vi "Example Circular Buffer Map.vi"() -> ()   [LabVIEW 2013]
uses:
  VariantBuffer/VariantBuffer.lvclass
  VariantBufferMap/VariantBufferMap.lvclass
panel:
  out "error out":errorcluster
  in  "preview count (-1: all)":i32=5
  out "found":bool
  out "elements":variant[](array[variant])
  in  "Buffer Name":string(combo)
  # "Select the Buffer to Preview"
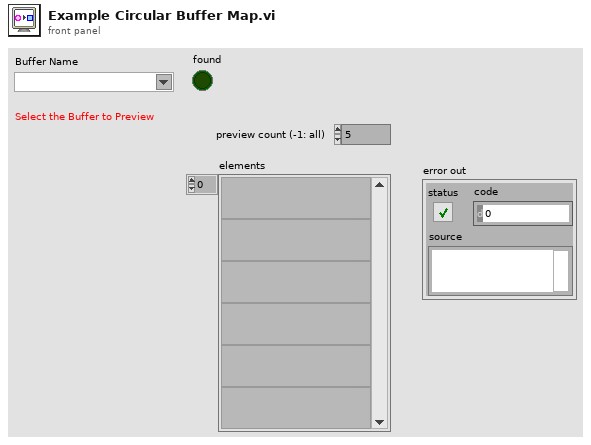
[diagram p1: front panel]
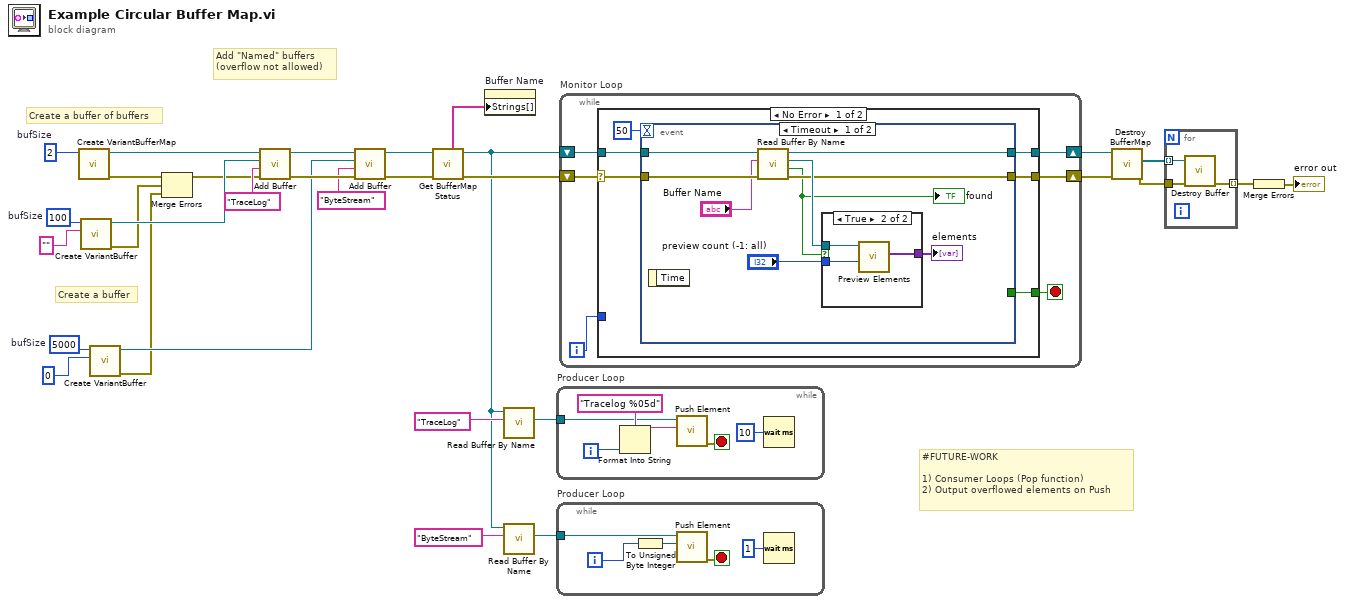
[diagram p0: block diagram]
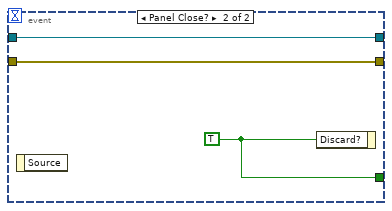
[diagram p3: hidden frame]
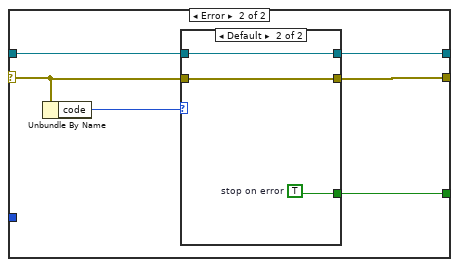
[diagram p4: hidden frame]
diagram:
  w8 = 5000  # bufSize
  w29 = 2  # bufSize
  w31 = 100  # bufSize
  # "#FUTURE-WORK\n\n1) Consumer Loops (Pop function)\n2) Output overflowed elements on Push"
  # "Create a buffer"
  # "Add \"Named\" buffers\n(overflow not allowed)"
  # "Create a buffer of buffers"
  n1 = call "Create VariantBufferMap.vi"("bufSize"=w29) -> ("error out"=w22:errorcluster, "BufferMap"=w23:refnum<data-value>)  [unwired: 9 in]
  n2 = call "Create VariantBuffer.vi"("default"="", "bufSize"=w31) -> ("error out"=w21:errorcluster, "Buffer"=w27:refnum<data-value>)  [unwired: 8 in]
  n3 = call "Create VariantBuffer.vi"("default"=u8 0, "bufSize"=w8) -> ("error out"=w4:errorcluster, "Buffer"=w6:refnum<data-value>)  [unwired: 8 in]
  n4 = Merge Errors(w22, w21, w4) -> (w20:errorcluster)
  n5 = call "Add Buffer.vi"("error in"=w20, "Name"="TraceLog", "Buffer"=w27, "BufferMap in"=w23) -> ("error out"=w11:errorcluster, "BufferMap"=w13:refnum<data-value>)  [unwired: 6 in]
  n6 = call "Add Buffer.vi"("error in"=w11, "Name"="ByteStream", "Buffer"=w6, "BufferMap in"=w13) -> ("error out"=w10:errorcluster, "BufferMap"=w12:refnum<data-value>)  [unwired: 6 in]
  n7 = call "Get BufferMap Status.vi"("error in"=w10, "BufferMap in"=w12) -> ("error out"=w17:errorcluster, "BufferMap"=w14:refnum<data-value>, "Names"=w18:string[])  [unwired: 4 in, 3 out]
  n8 = property on="Buffer Name" class="CmbBox"("Strings[]"=w18) -> ()  [unwired: 2 in, 2 out]
  n9 = call "Read Buffer By Name.vi"("Name"="TraceLog", "BufferMap in"=w14) -> ("Buffer"=w24:refnum<data-value>)  [unwired: 6 in, 3 out]
  n10 = call "Read Buffer By Name.vi"("Name"="ByteStream", "BufferMap in"=w14) -> ("Buffer"=w16:refnum<data-value>)  [unwired: 6 in, 3 out]
  n11 = while "Producer Loop" {
    tunnel: w24 -> [w34]
    i -> [w36]
    stop <- w32 stop-if-true
    n12 = Format Into String(format string="Tracelog %05d", w36) -> (resulting string=w33:string)  [unwired: 2 in, 1 out]
    n13 = call "Push Element.vi"("element"=w33, "Buffer in"=w34) -> ("error out"=w32:errorcluster)  [unwired: 8 in, 1 out]
    n14 = Wait (ms)(milliseconds to wait=u32 10) -> ()  [unwired: 1 out]
  }
  n15 = while "Producer Loop" {
    tunnel: w16 -> [w41]
    i -> [w38]
    stop <- w40 stop-if-true
    n16 = To Unsigned Byte Integer(number=w38) -> (unsigned 8bit integer=w39:u8)
    n17 = call "Push Element.vi"("element"=w39, "Buffer in"=w41) -> ("error out"=w40:errorcluster)  [unwired: 8 in, 1 out]
    n18 = Wait (ms)(milliseconds to wait=u32 1) -> ()  [unwired: 1 out]
  }
  n19 = while "Monitor Loop" {
    shift-right: [w47] -> w26
    shift-left: w14 -> [w48]
    shift-right: [w46] -> w19
    shift-left: w17 -> [w44]
    i -> [w43]
    stop <- w45 stop-if-true
    n20 = case shown="No Error" w44 {
      selector: w44 -> [w49 w71]
      tunnel: w48 -> [w53 w72]
      tunnel: [w52 w73] -> w47
      tunnel: [w51 w70] -> w46
      tunnel: [w50 w75] -> w45
      tunnel: w43 -> [_ _]
      frame No Error {
        n21 = event shown="[0] Timeout" {
          selector: _ -> [_ _]
          dyn-events: _ -> [_ _]
          timeout: 50 -> [_ _]
          tunnel: w53 -> [w63 w69]
          tunnel: [w62 w69] -> w52
          tunnel: [_ w68] -> w50
          tunnel: w49 -> [w60 w67]
          tunnel: [w59 w67] -> w51
          event Timeout {
            n22 = event-data() -> ()  [unwired: 1 in, 1 out]
            n23 = call "Read Buffer By Name.vi"("error in (no error)"=w60, "Name"="Buffer Name", "BufferMap in"=w63) -> ("error out"=w59:errorcluster, "found"=w57:bool, "Buffer"=w61:refnum<data-value>, "BufferMap"=w62:refnum<data-value>)  [unwired: 5 in]
            "found" <- w57
            n24 = case shown="True" w57 {
              tunnel: w61 -> [_ w66]
              tunnel: [_ w65] -> w56
              tunnel: "preview count (-1: all)" -> [_ w64]
              frame False {
              }
              frame True {
                n25 = call "Preview Elements.vi"("count (-1: all)"=w64, "ByteBuffer in"=w66) -> ("elements"=w65:variant[])  [unwired: 7 in, 2 out]
              }
            }
            "elements" <- w56
          }
          event Panel Close? {
            w68 = TRUE ("Discard?")
            n26 = event-data() -> ()  [unwired: 1 in, 1 out]
            n27 = event-data("Discard?"=w68) -> ()  [unwired: 1 in, 1 out]
          }
        }
      }
      frame Error {
        n28 = Unbundle By Name(w71) -> ("code"=w74:i32)
        n29 = case shown="Default" w74 {
          tunnel: [_ w79] -> w75
          tunnel: [w76 w78] -> w73
          tunnel: w72 -> [w76 w78]
          tunnel: w71 -> [_ w77]
          tunnel: [_ w77] -> w70
          frame 0 {
            # "Handle Error\n& Continue"
          }
          frame Default {
            w79 = TRUE  # stop on error
          }
        }
      }
    }
  }
  n30 = call "Destroy BufferMap.vi"("error in"=w19, "Buffer"=w26) -> ("error out"=w3:errorcluster, "elements"=w30:refnum<data-value>[])  [unwired: 8 in]
  n31 = for {
    tunnel: w30 -> [w82] mode=indexing
    tunnel: w3 -> [w81]
    tunnel: [w80] -> w2 mode=indexing
    n32 = call "Destroy Buffer.vi"("error in"=w81, "Buffer"=w82) -> ("error out"=w80:errorcluster)  [unwired: 8 in, 1 out]
  }
  n33 = Merge Errors(w2) -> (→"error out":errorcluster)
